vi "Create NI 9437 - Counter Input PWM.vi"(8 "error in":errorcluster, 11 "channel settings":T1[](array[typedef])) -> (0 "error out":errorcluster, 3 "NI 9437 out":refnum<class "NI 9437.lvclass">)   [LabVIEW 2020, in "Scan Engine Scripting.lvlib" / "NI 9437.lvclass"]
doc: "Creates and configures an instance of a NI-9437 counter input Pulse Width Modulation (PWM) module that can be used to set a slot in a Scan Engine custom device chassis."
uses:
  NI 9437.lvclass
  Mode Classes/Controls/counter input pwm channel settings.ctl
  Channel Classes/PWM Input Channel/Measurement Type.ctl
  Mode Classes/Counter Input PWM Mode/Counter Input PWM Mode.lvclass
  C:/jenkins/workspace/ercat-custom-device_release_20.4/Custom Device Source/Scripting/Modules/Mode Classes/Mode/Mode.lvclass
  00c94b37-37fe-4450-80ce-a87fb43ff01e.vi
  Channel Classes/PWM Input Channel/PWM Input Channel.lvclass
  Scan Engine Scripting.lvlib
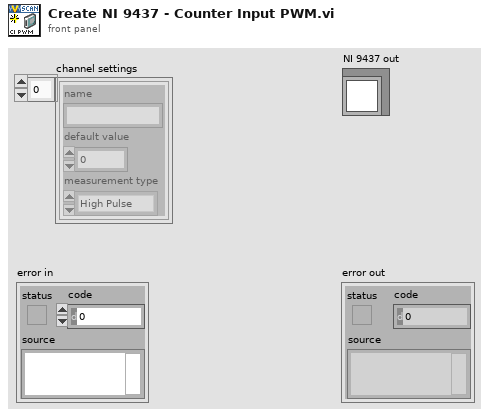
[diagram p1: front panel]
types:
  T1 = typedef "Scan Engine Scripting.lvlib/counter input pwm channel settings.ctl" = cluster{"name":string, "default value":dbl, "measurement type":T2}
  T2 = typedef "Scan Engine Scripting.lvlib/PWM Input Channel.lvclass/Measurement Type.ctl" = enum16{"High Pulse", "Low Pulse", "Most Recent"}
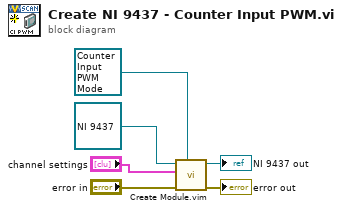
[diagram p0: block diagram]
diagram:
  n1 = call "Create Module.vim"("mode"=refnum<class "Counter Input PWM Mode.lvclass"> refnum ("Scan Engine Scripting.lvlib:Counter Input PWM Mode.lvclass"), "error in"="error in", "channel settings"="channel settings", "module in"=refnum<class "NI 9437.lvclass"> refnum ("Scan Engine Scripting.lvlib:NI 9437.lvclass")) -> ("error out"=→"error out":errorcluster, "module out"=→"NI 9437 out":refnum<class "NI 9437.lvclass">)  [unwired: 6 in]
